vi "DecodeAvs47bConfiguration.vi"(2 "RXSTR":string="000000000110010000000011000111101001100101010000") -> (5 "INPUT OUT":u16(ring) items=["ZERO", "MEAS", "CAL"], 6 "CHANNEL OUT":u16(ring) items=["CH0", "CH1", "CH2", "CH3", "CH4", "CH5", "CH6", "CH7"], 7 "RANGE OUT":u16(ring) items=["NO RANGE", "2 Ohms", "20 Ohms", "200 Ohms", "2 kOhms", "20 kOhms", "200 kOhms", "2 MOhms"], 8 "DISPLAY OUT":u16(ring) items=["R", "DR", "ADJ REF", "REFERENCE", "EXC VOLT", "530A HEAT V", "530A HEAT I", "530A SET PT"], 9 "EXCITATION OUT":u16(ring) items=["NO EXCITATION", "3 uV", "10uV", "30uV", "100uV", "300uV", "1mV", "3mV"])   [LabVIEW 2021]
doc: "Used by ReadAvs47b.vi"
panel:
  out "2  bits":u16
  out "8 bits":u16
  out "16 bits":u16
  # "Decode AVS-47B Configuration  rev 3.0"
  # "DecodeAvs47bConfiguration.vi"
  # "(input to this  VI is the received string from AVS-47B)"
  # "Extracts the complete configuration of the AVS-47B from\nits Picobus response string.  This VI is especially useful when\nthe bridge is in local mode while the computer only collects\nand handles the results."
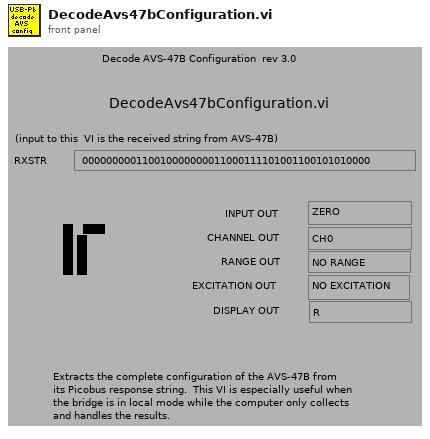
[diagram p1: front panel]
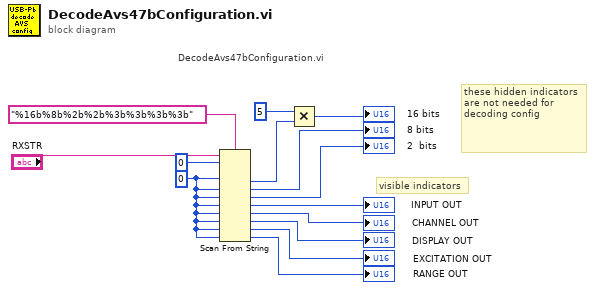
[diagram p0: block diagram]
diagram:
  w6 = u16 0
  # "DecodeAvs47bConfiguration.vi"
  # "visible indicators"
  # "these hidden indicators\nare not needed for decoding config"
  n1 = Scan From String(format string="%16b%8b%2b%2b%3b%3b%3b%3b", input string="RXSTR", initial scan location=u16 0, default 1=w6, default 2=w6, default 3=w6, default 4=w6, default 5=w6, default 6=w6, default 7=w6, default 8=w6) -> (output 1=w9:u16, output 2=→"8 bits":u16, output 3=→"2  bits":u16, output 4=→"INPUT OUT":u16, output 5=→"CHANNEL OUT":u16, output 6=→"DISPLAY OUT":u16, output 7=→"EXCITATION OUT":u16, output 8=→"RANGE OUT":u16)  [unwired: 1 in, 3 out]
  n2 = Multiply(x=u16 5, y=w9) -> (x*y=→"16 bits":u16)
